vi "fit std deviation away from crossing.vi"() -> ()   [LabVIEW 2016]
uses:
  <vilib>/Analysis/NI_AALPro.lvlib
panel:
  in  "trion 0823":cluster{dbl[], dbl[]}(graph)={[-8.95, -8.9, -8.85, -8.8, -8.75, -8.7, -8.65, -8.6, -8.55, -8.5, -8.45, -8.4, -8.35, -8.3, -8.25, -8.2, -8.15, -8.1, -8.05, -8.0, -7.95, -7.9, -7.85, -7.8, -7.75, -7.7, -7.65, -7.6, -7.55, -7.5, -7.45, -7.4, -7.35, -7.3, -7.25, -7.2, -7.15, -7.1, -7.05, -7.0, -6.949999999999999, -6.9, -6.85, -6.8, -6.75, -6.699999999999999, -6.65, -6.6, -6.55, -6.5, -6.449999999999999, -6.4, -6.35, -6.3, -6.25, -6.199999999999999, -6.15, -6.1, -6.05, -6.0, -5.949999999999999, -5.9, -5.85, -5.8, -5.75, -5.699999999999999, -5.65, -5.6, -5.55, -5.5, -5.449999999999999, -5.4, -5.35, -5.3], [0.04218999316467269, 0.04075199693938387, 0.04045283953059347, 0.03909051713328811, 0.037793448361722166, 0.03700068877459801, 0.0349324870970816, 0.03331217035816056, 0.0314909975356083, 0.03177403817584393, 0.02932753418691237, 0.02700804360768333, 0.02633178372115984, 0.03158113527106622, 0.02404551812182299, 0.022966818279259782, 0.021544994547486335, 0.0201169542942942, 0.01809988004003692, 0.017760337302324385, 0.015375826856933264, 0.015540451766346065, 0.01238254363365873, 0.01197793465386566, 0.01469140459758915, 0.011482438161231933, 0.011788518454902782, 0.0075208800302881615, 0.006609982768005348, 0.00868818688284046, 0.024210964202999095, 0.007288780850591874, 0.005007141026599192, 0.004244529981348508, 0.0027613068855327823, 1.08161430489982e-05, 0.0010862040019150913, 0.0010631417935129965, 0.004028837450315436, 0.0047069012690502225, 0.004525374955101665, 0.0008401724303967557, 0.003085904761832927, 0.002562505713076739, 0.0056535990499483645, 0.0023852254614874185, 0.002213050416617493, 0.0017981545630226094, 0.0026565662723808015, 0.00701627922628342, 0.009872116712613831, 0.011181058488079465, 0.01450183683233224, 0.01877042916919371, 0.019067143968683444, 0.015361077969213613, 0.022103829165370705, 0.022967807128503055, 0.023555243878749584, 0.025824536320352004, 0.02805065095889145, 0.027625440930324586, 0.029289172090061284, 0.031216530697626355, 0.03209095805188397, 0.03420267331879509, 0.035277756275320954, 0.03615351375849655, 0.0368454478183709, 0.044505664258700436, 0.03960154744342885, 0.04539023795135439, 0.04216822235434108, 0.040561394374812064]}
  in  "right length":i32=75
  in  "right index":i32=15
  in  "left length":i32=75
  in  "left index":i32
  out "pair 3":cluster{dbl[], "Best Linear Fit":dbl[]}[](graph)=[{[-8.95, -8.9, -8.85, -8.8, -8.75, -8.7, -8.65, -8.6, -8.55, -8.5, -8.45, -8.4, -8.35, -8.3, -8.25, -8.2, -8.15, -8.1, -8.05, -8.0, -7.95, -7.9, -7.85, -7.8, -7.75, -7.7, -7.65, -7.6, -7.55, -7.5, -7.45, -7.4, -7.35, -7.3, -7.25, -7.2, -7.15, -7.1, -7.05, -7.0, -6.949999999999999, -6.9, -6.85, -6.8, -6.75, -6.699999999999999, -6.65, -6.6, -6.55, -6.5, -6.449999999999999, -6.4, -6.35, -6.3, -6.25, -6.199999999999999, -6.15, -6.1, -6.05, -6.0, -5.949999999999999, -5.9, -5.85, -5.8, -5.75, -5.699999999999999, -5.65, -5.6, -5.55, -5.5, -5.449999999999999, -5.4, -5.35, -5.3], "Best Linear Fit"=[0.04218999316467269, 0.04075199693938387, 0.04045283953059347, 0.03909051713328811, 0.037793448361722166, 0.03700068877459801, 0.0349324870970816, 0.03331217035816056, 0.0314909975356083, 0.03177403817584393, 0.02932753418691237, 0.02700804360768333, 0.02633178372115984, 0.03158113527106622, 0.02404551812182299, 0.022966818279259782, 0.021544994547486335, 0.0201169542942942, 0.01809988004003692, 0.017760337302324385, 0.015375826856933264, 0.015540451766346065, 0.01238254363365873, 0.01197793465386566, 0.01469140459758915, 0.011482438161231933, 0.011788518454902782, 0.0075208800302881615, 0.006609982768005348, 0.00868818688284046, 0.024210964202999095, 0.007288780850591874, 0.005007141026599192, 0.004244529981348508, 0.0027613068855327823, 1.08161430489982e-05, 0.0010862040019150913, 0.0010631417935129965, 0.004028837450315436, 0.0047069012690502225, 0.004525374955101665, 0.0008401724303967557, 0.003085904761832927, 0.002562505713076739, 0.0056535990499483645, 0.0023852254614874185, 0.002213050416617493, 0.0017981545630226094, 0.0026565662723808015, 0.00701627922628342, 0.009872116712613831, 0.011181058488079465, 0.01450183683233224, 0.01877042916919371, 0.019067143968683444, 0.015361077969213613, 0.022103829165370705, 0.022967807128503055, 0.023555243878749584, 0.025824536320352004, 0.02805065095889145, 0.027625440930324586, 0.029289172090061284, 0.031216530697626355, 0.03209095805188397, 0.03420267331879509, 0.035277756275320954, 0.03615351375849655, 0.0368454478183709, 0.044505664258700436, 0.03960154744342885, 0.04539023795135439, 0.04216822235434108, 0.040561394374812064]}, {[-8.95, -8.9, -8.85, -8.8, -8.75, -8.7, -8.65, -8.6, -8.55, -8.5, -8.45, -8.4, -8.35, -8.3, -8.25, -8.2, -8.15, -8.1, -8.05, -8.0, -7.95, -7.9, -7.85, -7.8, -7.75, -7.7, -7.65, -7.6, -7.55, -7.5, -7.45, -7.4, -7.35, -7.3, -7.25, -7.2, -7.15, -7.1, -7.05, -7.0, -6.949999999999999, -6.9, -6.85, -6.8, -6.75, -6.699999999999999, -6.65, -6.6, -6.55, -6.5], "Best Linear Fit"=[0.04312773853449364, 0.041796552028319306, 0.04046536552214494, 0.039134179015970605, 0.03780299250979621, 0.03647180600362185, 0.03514061949744751, 0.03380943299127312, 0.03247824648509878, 0.03114705997892442, 0.029815873472750026, 0.02848468696657569, 0.027153500460401298, 0.02582231395422696, 0.024491127448052596, 0.023159940941878204, 0.021828754435703868, 0.020497567929529503, 0.019166381423355167, 0.017835194917180774, 0.01650400841100641, 0.015172821904832046, 0.013841635398657681, 0.012510448892483317, 0.011179262386308952, 0.009848075880134588, 0.008516889373960251, 0.007185702867785859, 0.005854516361611495, 0.00452332985543713, 0.0031921433492627938, 0.0018609568430884293, 0.0005297703369140372, -0.0008014161692602995, -0.002132602675434664, -0.0034637891816090283, -0.004794975687783393, -0.006126162193957757, -0.0074573487001321215]}, {[-7.2, -7.15, -7.1, -7.05, -7.0, -6.949999999999999, -6.9, -6.85, -6.8, -6.75, -6.699999999999999, -6.65, -6.6, -6.55, -6.5, -6.449999999999999, -6.4, -6.35, -6.3, -6.25, -6.199999999999999, -6.15, -6.1, -6.05, -6.0, -5.949999999999999, -5.9, -5.85, -5.8, -5.75, -5.699999999999999, -5.65, -5.6, -5.55, -5.5, -5.449999999999999, -5.4, -5.35, -5.3], "Best Linear Fit"=[-0.007578397138169823, -0.0061977000021991024, -0.0048170028662283815, -0.0034363057302576605, -0.0020556085942869395, -0.0006749114583161908, 0.0007057856776545024, 0.002086482813625251, 0.003467179949595972, 0.004847877085566693, 0.006228574221537414, 0.007609271357508107, 0.008989968493478856, 0.010370665629449577, 0.011751362765420298, 0.013132059901391047, 0.01451275703736174, 0.01589345417333246, 0.017274151309303182, 0.018654848445273903, 0.02003554558124465, 0.021416242717215345, 0.022796939853186093, 0.024177636989156814, 0.025558334125127508, 0.026939031261098256, 0.02831972839706895, 0.029700425533039698, 0.03108112266901042, 0.03246181980498114, 0.03384251694095189, 0.03522321407692258, 0.0366039112128933, 0.037984608348864024, 0.039365305484834745, 0.040746002620805494, 0.04212669975677619, 0.043507396892746936, 0.04488809402871766]}]
  out "pair 2":cluster{dbl[], "Best Linear Fit":dbl[]}[](graph)=[{[-8.95, -8.9, -8.85, -8.8, -8.75, -8.7, -8.65, -8.6, -8.55, -8.5, -8.45, -8.4, -8.35, -8.3, -8.25, -8.2, -8.15, -8.1, -8.05, -8.0, -7.95, -7.9, -7.85, -7.8, -7.75, -7.7, -7.65, -7.6, -7.55, -7.5, -7.45, -7.4, -7.35, -7.3, -7.25, -7.2, -7.15, -7.1, -7.05, -7.0, -6.949999999999999, -6.9, -6.85, -6.8, -6.75, -6.699999999999999, -6.65, -6.6, -6.55, -6.5, -6.449999999999999, -6.4, -6.35, -6.3, -6.25, -6.199999999999999, -6.15, -6.1, -6.05, -6.0, -5.949999999999999, -5.9, -5.85, -5.8, -5.75, -5.699999999999999, -5.65, -5.6, -5.55, -5.5, -5.449999999999999, -5.4, -5.35, -5.3], "Best Linear Fit"=[0.04218999316467269, 0.04075199693938387, 0.04045283953059347, 0.03909051713328811, 0.037793448361722166, 0.03700068877459801, 0.0349324870970816, 0.03331217035816056, 0.0314909975356083, 0.03177403817584393, 0.02932753418691237, 0.02700804360768333, 0.02633178372115984, 0.03158113527106622, 0.02404551812182299, 0.022966818279259782, 0.021544994547486335, 0.0201169542942942, 0.01809988004003692, 0.017760337302324385, 0.015375826856933264, 0.015540451766346065, 0.01238254363365873, 0.01197793465386566, 0.01469140459758915, 0.011482438161231933, 0.011788518454902782, 0.0075208800302881615, 0.006609982768005348, 0.00868818688284046, 0.024210964202999095, 0.007288780850591874, 0.005007141026599192, 0.004244529981348508, 0.0027613068855327823, 1.08161430489982e-05, 0.0010862040019150913, 0.0010631417935129965, 0.004028837450315436, 0.0047069012690502225, 0.004525374955101665, 0.0008401724303967557, 0.003085904761832927, 0.002562505713076739, 0.0056535990499483645, 0.0023852254614874185, 0.002213050416617493, 0.0017981545630226094, 0.0026565662723808015, 0.00701627922628342, 0.009872116712613831, 0.011181058488079465, 0.01450183683233224, 0.01877042916919371, 0.019067143968683444, 0.015361077969213613, 0.022103829165370705, 0.022967807128503055, 0.023555243878749584, 0.025824536320352004, 0.02805065095889145, 0.027625440930324586, 0.029289172090061284, 0.031216530697626355, 0.03209095805188397, 0.03420267331879509, 0.035277756275320954, 0.03615351375849655, 0.0368454478183709, 0.044505664258700436, 0.03960154744342885, 0.04539023795135439, 0.04216822235434108, 0.040561394374812064]}, {[-8.85, -8.8, -8.75, -8.7, -8.65, -8.6, -8.55, -8.5, -8.45, -8.4, -8.35, -8.3, -8.25, -8.2, -8.15, -8.1, -8.05], "Best Linear Fit"=[0.04045283953059347, 0.03909051713328811, 0.037793448361722166, 0.03700068877459801, 0.0349324870970816, 0.03331217035816056, 0.0314909975356083, 0.03177403817584393, 0.02932753418691237, 0.02700804360768333, 0.02633178372115984, 0.03158113527106622, 0.02404551812182299, 0.022966818279259782, 0.021544994547486335, 0.0201169542942942, 0.01809988004003692]}, {[-8.85, -8.8, -8.75, -8.7, -8.65, -8.6, -8.55, -8.5, -8.45, -8.4, -8.35, -8.3, -8.25, -8.2, -8.15, -8.1, -8.05], "Best Linear Fit"=[0.04046536552214494, 0.039134179015970605, 0.03780299250979621, 0.03647180600362185, 0.03514061949744751, 0.03380943299127312, 0.03247824648509878, 0.03114705997892442, 0.029815873472750026, 0.02848468696657569, 0.027153500460401298, 0.02582231395422696, 0.024491127448052596, 0.023159940941878204, 0.021828754435703868, 0.020497567929529503, 0.019166381423355167]}, {[-6.1, -6.05, -6.0, -5.949999999999999, -5.9, -5.85, -5.8, -5.75, -5.699999999999999, -5.65], "Best Linear Fit"=[0.022967807128503055, 0.023555243878749584, 0.025824536320352004, 0.02805065095889145, 0.027625440930324586, 0.029289172090061284, 0.031216530697626355, 0.03209095805188397, 0.03420267331879509, 0.035277756275320954]}, {[-6.1, -6.05, -6.0, -5.949999999999999, -5.9, -5.85, -5.8, -5.75, -5.699999999999999, -5.65], "Best Linear Fit"=[0.022796939853186093, 0.024177636989156814, 0.025558334125127508, 0.026939031261098256, 0.02831972839706895, 0.029700425533039698, 0.03108112266901042, 0.03246181980498114, 0.03384251694095189, 0.03522321407692258]}]
  in  "length 2":i32=10
  in  "index 2":i32=57
  in  "length":i32=17
  in  "index":i32=2
  in  "pair":cluster{dbl[], dbl[]}(graph)={[-8.95, -8.9, -8.85, -8.8, -8.75, -8.7, -8.65, -8.6, -8.55, -8.5, -8.45, -8.4, -8.35, -8.3, -8.25, -8.2, -8.15, -8.1, -8.05, -8.0, -7.95, -7.9, -7.85, -7.8, -7.75, -7.7, -7.65, -7.6, -7.55, -7.5, -7.45, -7.4, -7.35, -7.3, -7.25, -7.2, -7.15, -7.1, -7.05, -7.0, -6.949999999999999, -6.9, -6.85, -6.8, -6.75, -6.699999999999999, -6.65, -6.6, -6.55, -6.5, -6.449999999999999, -6.4, -6.35, -6.3, -6.25, -6.199999999999999, -6.15, -6.1, -6.05, -6.0, -5.949999999999999, -5.9, -5.85, -5.8, -5.75, -5.699999999999999, -5.65, -5.6, -5.55, -5.5, -5.449999999999999, -5.4, -5.35, -5.3], [0.04218999316467269, 0.04075199693938387, 0.04045283953059347, 0.03909051713328811, 0.037793448361722166, 0.03700068877459801, 0.0349324870970816, 0.03331217035816056, 0.0314909975356083, 0.03177403817584393, 0.02932753418691237, 0.02700804360768333, 0.02633178372115984, 0.03158113527106622, 0.02404551812182299, 0.022966818279259782, 0.021544994547486335, 0.0201169542942942, 0.01809988004003692, 0.017760337302324385, 0.015375826856933264, 0.015540451766346065, 0.01238254363365873, 0.01197793465386566, 0.01469140459758915, 0.011482438161231933, 0.011788518454902782, 0.0075208800302881615, 0.006609982768005348, 0.00868818688284046, 0.024210964202999095, 0.007288780850591874, 0.005007141026599192, 0.004244529981348508, 0.0027613068855327823, 1.08161430489982e-05, 0.0010862040019150913, 0.0010631417935129965, 0.004028837450315436, 0.0047069012690502225, 0.004525374955101665, 0.0008401724303967557, 0.003085904761832927, 0.002562505713076739, 0.0056535990499483645, 0.0023852254614874185, 0.002213050416617493, 0.0017981545630226094, 0.0026565662723808015, 0.00701627922628342, 0.009872116712613831, 0.011181058488079465, 0.01450183683233224, 0.01877042916919371, 0.019067143968683444, 0.015361077969213613, 0.022103829165370705, 0.022967807128503055, 0.023555243878749584, 0.025824536320352004, 0.02805065095889145, 0.027625440930324586, 0.029289172090061284, 0.031216530697626355, 0.03209095805188397, 0.03420267331879509, 0.035277756275320954, 0.03615351375849655, 0.0368454478183709, 0.044505664258700436, 0.03960154744342885, 0.04539023795135439, 0.04216822235434108, 0.040561394374812064]}
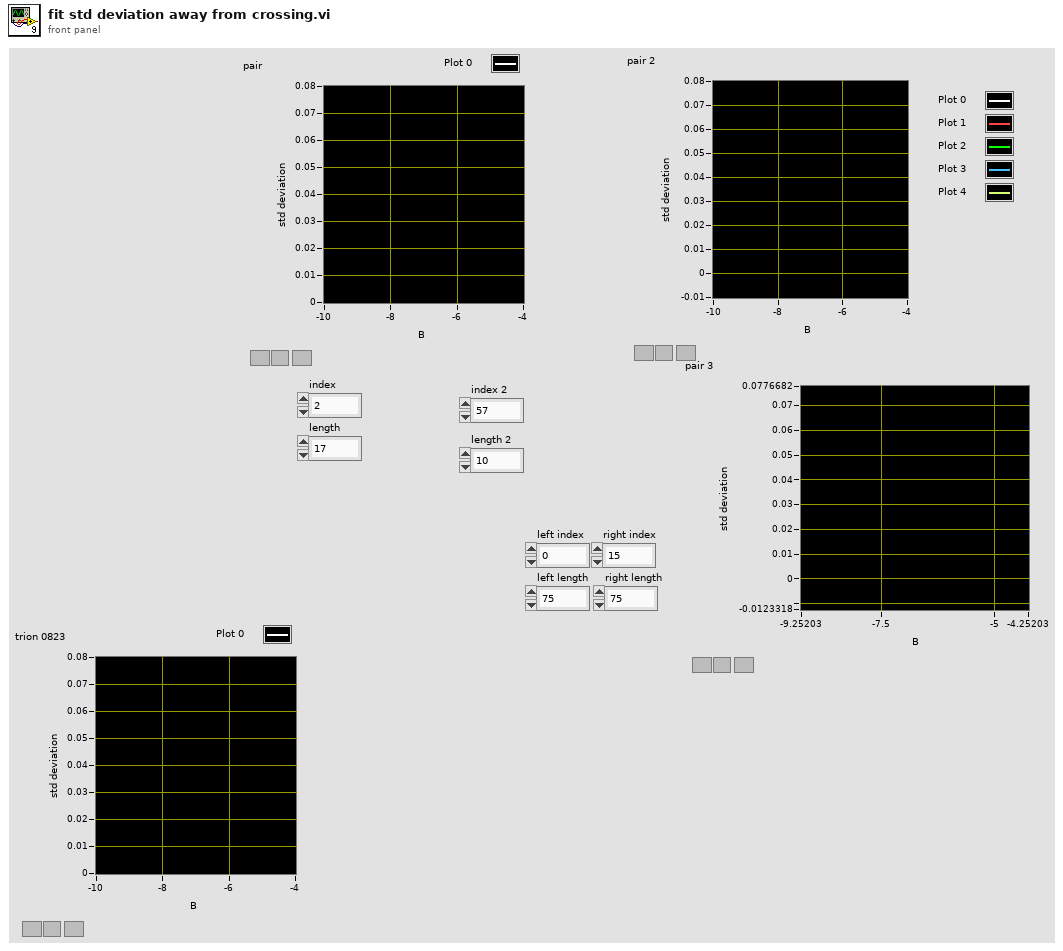
[diagram p1: front panel]
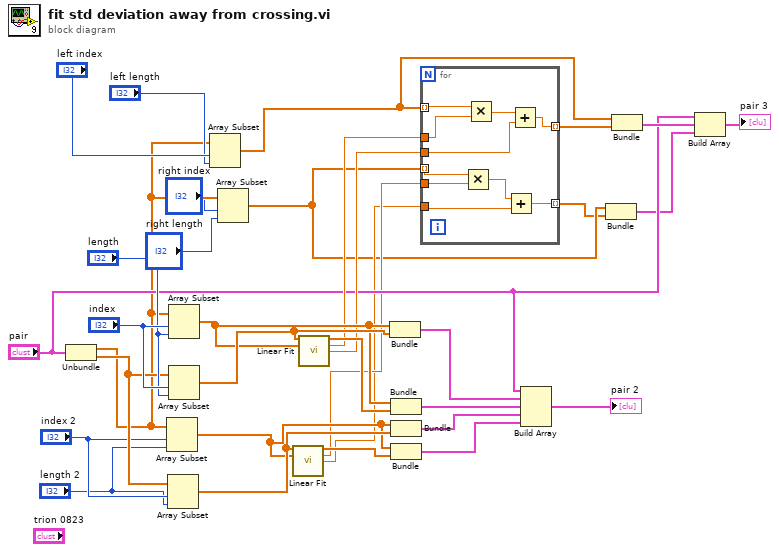
[diagram p0: block diagram]
diagram:
  n1 = Unbundle("pair") -> (w9:dbl[], w31:dbl[])
  n2 = Array Subset(array=w9, index="index 2", length="length 2") -> (w23:dbl[])
  n3 = Array Subset(array=w31, index="index 2", length="length 2") -> (w25:dbl[])
  n4 = Array Subset(array=w9, index="index", length="length") -> (w26:dbl[])
  n5 = Array Subset(array=w31, index="index", length="length") -> (w28:dbl[])
  n6 = Array Subset(array=w9, index="left index", length="left length") -> (w12:dbl[])
  n7 = Array Subset(array=w9, index="right index", length="right length") -> (w5:dbl[])
  n8 = call <vilib>:"Linear Fit.vi"("Y"=w25, "X"=w23) -> ("Best Linear Fit"=w24:dbl[], "slope"=w7:dbl, "intercept"=w6:dbl)  [unwired: 9 in, 2 out]
  n9 = call <vilib>:"Linear Fit.vi"("Y"=w28, "X"=w26) -> ("Best Linear Fit"=w27:dbl[], "slope"=w15:dbl, "intercept"=w14:dbl)  [unwired: 9 in, 2 out]
  n10 = Bundle(w26, w28) -> (w22:cluster{dbl[], dbl[]})  [unwired: 1 in]
  n11 = Bundle(w26, "Best Linear Fit"=w27) -> (w21:cluster{dbl[], "Best Linear Fit":dbl[]})  [unwired: 1 in]
  n12 = Bundle(w23, w25) -> (w20:cluster{dbl[], dbl[]})  [unwired: 1 in]
  n13 = Bundle(w23, "Best Linear Fit"=w24) -> (w19:cluster{dbl[], "Best Linear Fit":dbl[]})  [unwired: 1 in]
  n14 = for {
    tunnel: w12 -> [w43] mode=indexing
    tunnel: w15 -> [w42]
    tunnel: w14 -> [w40]
    tunnel: [w39] -> w13 mode=indexing
    tunnel: w5 -> [w38] mode=indexing
    tunnel: w7 -> [w37]
    tunnel: w6 -> [w35]
    tunnel: [w34] -> w4 mode=indexing
    n15 = Multiply(x=w38, y=w37) -> (x*y=w36:dbl)
    n16 = Multiply(x=w43, y=w42) -> (x*y=w41:dbl)
    n17 = Add(x=w36, y=w35) -> (x+y=w34:dbl)
    n18 = Add(x=w41, y=w40) -> (x+y=w39:dbl)
  }
  n19 = Build Array("pair", w22, w21, w20, w19) -> (→"pair 2":cluster{dbl[], "Best Linear Fit":dbl[]}[])
  n20 = Bundle(w5, w4) -> (w3:cluster{dbl[], dbl[]})  [unwired: 1 in]
  n21 = Bundle(w12, w13) -> (w11:cluster{dbl[], dbl[]})  [unwired: 1 in]
  n22 = Build Array("pair", w11, w3) -> (→"pair 3":cluster{dbl[], dbl[]}[])
